vi "Panel.vi"(11 "GWebAppArrayPanel in":refnum<class "GWebAppArrayPanel.lvclass">) -> ()   [LabVIEW 2020, in "PicoG-App.lvlib" / "GWebAppArrayPanel.lvclass"]
uses:
  GWebAppArrayPanel.lvclass
  C:/Program Files (x86)/National Instruments/LabVIEW 2020/vi.lib/IlluminatedG/IG OOPanel/OOPanel/Panel/Panel.lvclass
  <vilib>/IlluminatedG/IG OOPanel/OOPanel/Panel/Basic UI State.ctl
  GWebAppArrayPanel.lvclass/GWebAppArrayPanel.ctl
  ViaApp/ViaApp.lvclass
  <vilib>/IlluminatedG/IG OOPanel/OOPanel/Panel/Panel.lvclass
  <vilib>/IlluminatedG/IG OOPanel/OOPanel/OOPanel.lvlib
panel:
  out "Last Update":timestamp
  out "Updated":string
  out "Name":string
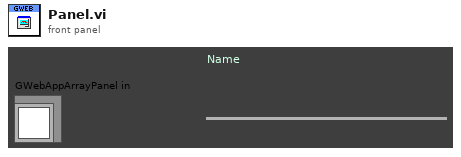
[diagram p1: front panel]
types:
  T1 = typedef "OOPanel.lvlib/Panel.lvclass/Basic UI State.ctl" = enum16{"Init", "Run", "Close"}
  T2 = typedef "PicoG-App.lvlib/GWebAppArrayPanel.lvclass/Inbound Events.ctl" = cluster{"Set Highlighted":refnum<user-event>, "App Updated":refnum<user-event>, "Remove App":refnum<user-event>}
  T3 = typedef "OOPanel.lvlib/Panel.lvclass/Panel Events.ctl" = cluster{"Visbility":refnum<user-event>, "Close":refnum<user-event>}
  T4 = typedef "PicoG-App.lvlib/GWebAppArrayPanel.lvclass/Ref Data.ctl" = cluster{"App":refnum<class "ViaApp.lvclass">}
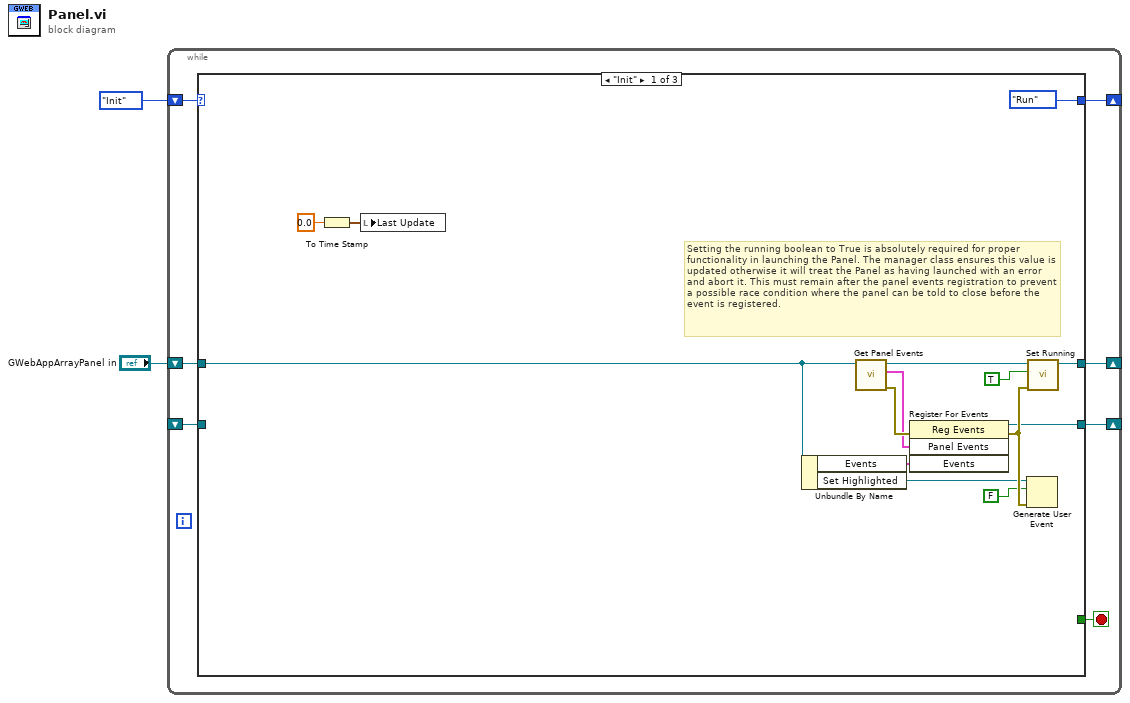
[diagram p0: block diagram]
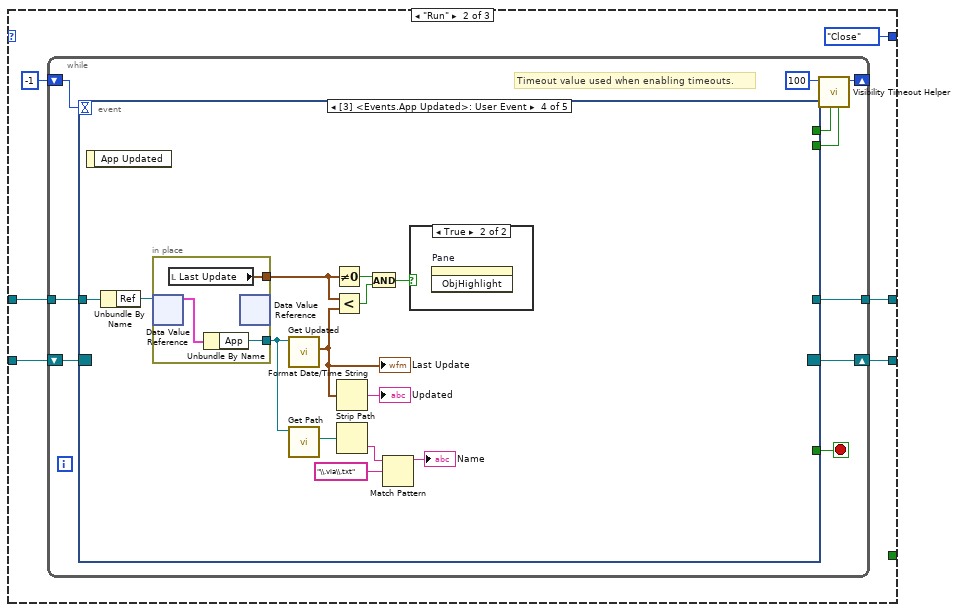
[diagram p2: hidden frame]
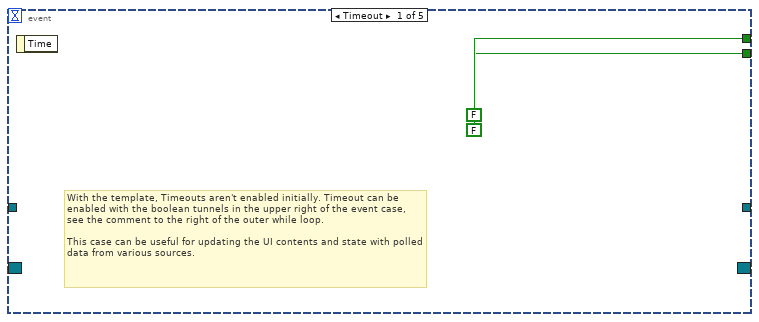
[diagram p3: hidden frame]
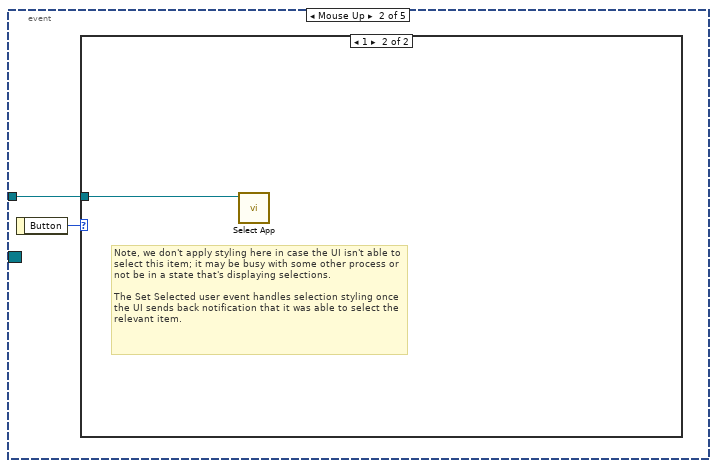
[diagram p4: hidden frame]
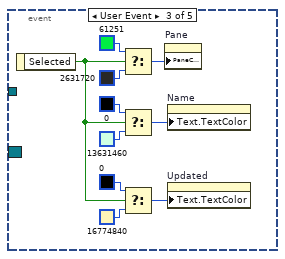
[diagram p6: hidden frame]
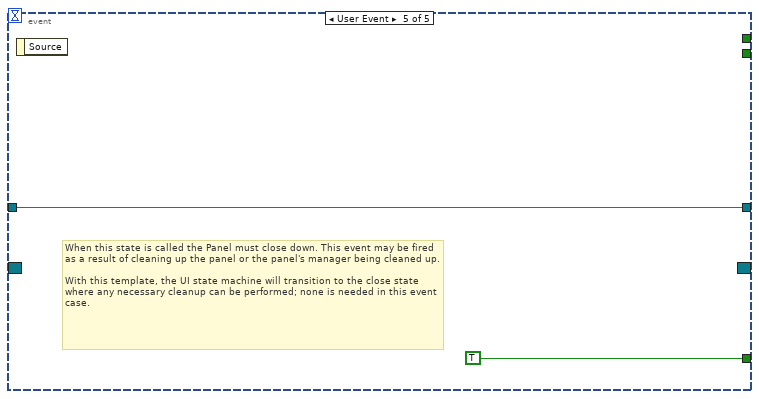
[diagram p8: hidden frame]
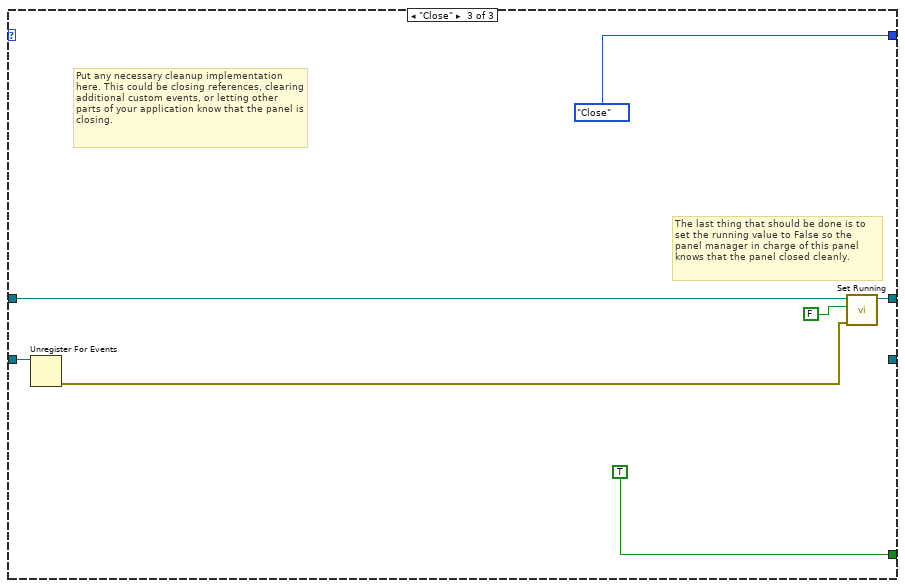
[diagram p9: hidden frame]
diagram:
  n1 = while {
    shift-right: [w8] -> _
    shift-left: _ -> [w9]
    shift-right: [w6] -> _
    shift-left: Basic_UI_State."Init" ("Basic UI State") -> [w7]
    shift-right: [w4] -> _
    shift-left: "GWebAppArrayPanel in" -> [w3]
    stop <- w5 stop-if-true
    n2 = case shown="\"Init\"" w7 {
      tunnel: w9 -> [_ w29 w75]
      tunnel: [w17 w27 _] -> w8
      tunnel: [Basic_UI_State."Run" ("Basic UI State") Basic_UI_State."Close" ("Basic UI State") Basic_UI_State."Close" ("Basic UI State")] -> w6
      tunnel: [_ _ TRUE] -> w5
      tunnel: [w16 w24 w73] -> w4
      tunnel: w3 -> [w15 w25 w74]
      frame "Init" {
        # "Setting the running boolean to True is absolutely required for proper functionality in launching the Panel. The manager class ensures this value is updated otherwise it will treat the Panel as having launched with an error and abort it. This must remain after the panel events registration to prevent a possible race condition where the panel can be told to close before the event is registered."
        n3 = To Time Stamp(1:0.0) -> (0:w10:timestamp)
        n4 = local write "Last Update"(w10) -> ()
        n5 = Unbundle By Name(w15) -> ("Events"=w14:T2, "Set Highlighted"=w13:refnum<user-event>)
        n6 = call <vilib>:"Get Panel Events.vi"("Panel in"=w15) -> ("error out"=w22:errorcluster, "Panel Events"=w19:T3, "Panel out"=w20:refnum<class "GWebAppArrayPanel.lvclass">)  [unwired: 8 in]
        n7 = register-events(error in=w22, w19, w14) -> (reference out=w17:refnum<event-registration>, error out=w23:errorcluster)  [unwired: 1 in]
        n8 = Generate User Event(user event=w13, event data cluster=FALSE ("event data"), error in=w23) -> ()  [unwired: 1 in, 2 out]
        n9 = call <vilib>:"Set Running.vi"("error in (no error)"=w23, "Running"=TRUE, "Panel in"=w20) -> ("Panel out"=w16:refnum<class "GWebAppArrayPanel.lvclass">)  [unwired: 7 in, 1 out]
      }
      frame "Run" {
        n10 = while {
          shift-right: [w35] -> w27
          shift-left: w29 -> [w36]
          shift-right: [w38] -> _
          shift-left: -1 ("Timeout") -> [w37]
          tunnel: w25 -> [w31]
          tunnel: [w30] -> w24
          stop <- w32 stop-if-true
          # "Timeout value used when enabling timeouts."
          n11 = event shown="[3] <Events.App Updated>: User Event" {
            selector: w36 -> [_ _ _ _ _]
            dyn-events: [_ _ _ _ _] -> w35
            timeout: w37 -> [_ _ _ _ _]
            tunnel: [FALSE _ _ _ _] -> w34
            tunnel: [FALSE _ _ _ _] -> w33
            tunnel: [_ _ _ _ TRUE] -> w32
            tunnel: w31 -> [_ w42 _ w66 w71]
            tunnel: [_ _ _ _ w71] -> w30
            event Timeout {
              # "With the template, Timeouts aren't enabled initially. Timeout can be enabled with the boolean tunnels in the upper right of the event case, see the comment to the right of the outer while loop.\n\nThis case can be useful for updating the UI contents and state with polled data from various sources."
              n12 = event-data() -> ()  [unwired: 1 in, 1 out]
            }
            event Mouse Up {
              n13 = event-data() -> ("Button"=w43:u16)  [unwired: 1 in]
              n14 = case shown="1" w43 {
                tunnel: w42 -> [_ w44]
                frame Default {
                }
                frame 1 {
                  # "Note, we don't apply styling here in case the UI isn't able to select this item; it may be busy with some other process or not be in a state that's displaying selections.\n\nThe Set Selected user event handles selection styling once the UI sends back notification that it was able to select the relevant item."
                  n15 = call "Select App.vi"("GWebAppArrayPanel in"=w44) -> ()  [unwired: 9 in, 2 out]
                }
              }
            }
            event User Event {
              n16 = event-data() -> ("Selected"=w46:bool)  [unwired: 1 in]
              n17 = Select(t=u32 61251, s=w46, f=u32 2631720) -> (s? t:f=w52:u32)
              n18 = Select(t=u32 0, s=w46, f=u32 13631460) -> (s? t:f=w49:u32)
              n19 = Select(t=u32 0, s=w46, f=u32 16774840) -> (s? t:f=w45:u32)
              n20 = property on="Pane" class="Pane"("PaneColor"=w52) -> ()  [unwired: 2 in, 2 out]
              n21 = property on="Name" class="Str"("Text.TextColor"=w49) -> ()  [unwired: 2 in, 2 out]
              n22 = property on="Updated" class="Str"("Text.TextColor"=w45) -> ()  [unwired: 2 in, 2 out]
            }
            event User Event {
              n23 = event-data() -> ()  [unwired: 1 in, 1 out]
              n24 = Unbundle By Name(w66) -> ("Ref"=w67:refnum<data-value>)
              n25 = in-place {
                in-place-border: [w69] -> w65
                in-place-border: [w68] -> w63
                n26 = in-place-dvr #1(w67) -> (w70:T4)  [unwired: 1 out]
                n27 = local read "Last Update"() -> (w68:timestamp)
                n28 = Unbundle By Name(w70) -> ("App"=w69:refnum<class "ViaApp.lvclass">)
                n29 = in-place-dvr #1() -> ()  [unwired: 1 in, 2 out]
              }
              n30 = call "Get Updated.vi"("ViaApp in"=w65) -> ("Last Update"=w62:timestamp)  [unwired: 8 in, 2 out]
              "Last Update" <- w62
              n31 = call "Get Path.vi"("ViaApp in"=w65) -> ("Path"=w58:path)  [unwired: 8 in, 2 out]
              n32 = Not Equal To 0?(x=w63) -> (x != 0?=w61:bool)
              n33 = Less?(x=w63, y=w62) -> (x < y?=w60:bool)
              n34 = Format Date/Time String(seconds (now)=w62) -> (date/time string=→"Updated":string)  [unwired: 2 in]
              n35 = Strip Path(path=w58) -> (name=w57:string)  [unwired: 1 out]
              n36 = And(x=w61, y=w60) -> (x .and. y?=w59:bool)
              n37 = Match Pattern(string=w57, regular expression="\\.via\\.txt") -> (before substring=→"Name":string)  [unwired: 1 in, 3 out]
              n38 = case shown="True" w59 {
                frame False {
                }
                frame True {
                  n39 = invoke on="Pane" class="Pane" method="ObjHighlight"() -> ()  [unwired: 3 in, 3 out]
                }
              }
            }
            event User Event {
              # "When this state is called the Panel must close down. This event may be fired as a result of cleaning up the panel or the panel's manager being cleaned up.\n\nWith this template, the UI state machine will transition to the close state where any necessary cleanup can be performed; none is needed in this event case."
              n40 = event-data() -> ()  [unwired: 1 in, 1 out]
            }
          }
          n41 = call <vilib>:"Visibility Timeout Helper.vi"("Update?"=w33, "Use Timeout?"=w34, "Visible Timeout mS"=100) -> ("Timeout"=w38:i32)  [unwired: 8 in]
        }
      }
      frame "Close" {
        # "Put any necessary cleanup implementation here. This could be closing references, clearing additional custom events, or letting other parts of your application know that the panel is closing."
        # "The last thing that should be done is to set the running value to False so the panel manager in charge of this panel knows that the panel closed cleanly."
        n42 = Unregister For Events(event registration refnum=w75) -> (error out=w77:errorcluster)  [unwired: 1 in]
        n43 = call <vilib>:"Set Running.vi"("error in (no error)"=w77, "Running"=FALSE, "Panel in"=w74) -> ("Panel out"=w73:refnum<class "GWebAppArrayPanel.lvclass">)  [unwired: 7 in, 1 out]
      }
    }
  }
